vi "Write Startup Model-View Configuration.vi"(8 "Mediator":refnum<class "IMediator.lvclass">, 9 "Model":refnum<class "IModel.lvclass">, 10 "Startup View Configuration":refnum<class "IViewable.lvclass">, 11 "IViewModel In":refnum<class "IViewModel.lvclass">) -> (3 "IViewModel Out":refnum<class "IViewModel.lvclass">)   [LabVIEW 2015, in "IViewModel.lvlib" / "IViewModel.lvclass"]
doc: "<License>\nCopyright © 2017 Composed Systems, LLC | All rights reserved\nwww.composed.io\n\nAuthor: Ethan Stern <ethan.stern@composed.io>\n\nThis software is provided \"AS IS\" WITHOUT WARRANTIES, either express or implied, AND IS FOR EDUCATIONAL PURPOSES ONLY.\n</License>"
uses:
  IViewModel.lvclass
  IViewable/IViewable/IViewable.lvclass
  IModel/IModel/IModel.lvclass
  IMediator/IMediator/IMediator.lvclass
  IViewModel.lvclass/IViewModel.ctl
  IViewManager/IViewManager Messages/Launch Nested Views Msg/Launch Nested Views Msg.lvclass/Launch Nested Views Msg.ctl
  IViewManager/IViewManager/IViewManager.lvclass/IViewManager.ctl
  IViewManager/IViewManager Messages/Launch Nested Views Msg/Launch Nested Views Msg.lvclass
  IViewManager/IViewManager/IViewManager.lvclass
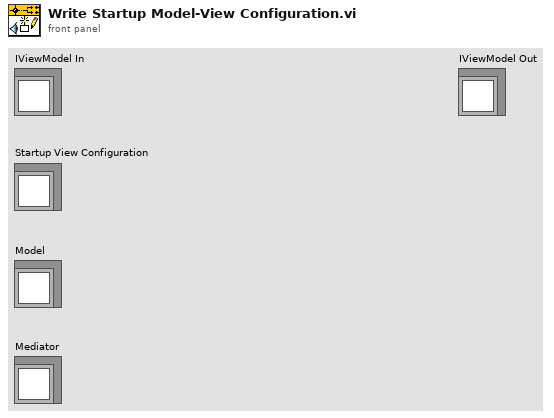
[diagram p1: front panel]
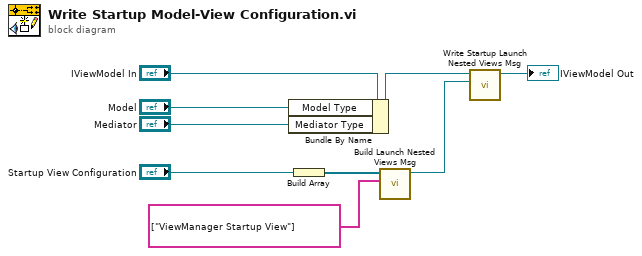
[diagram p0: block diagram]
diagram:
  n1 = Bundle By Name(cluster="IViewModel In", "Model Type"="Model", "Mediator Type"="Mediator") -> (w3:refnum<class "IViewModel.lvclass">)
  n2 = Build Array("Startup View Configuration") -> (w7:refnum<class "IViewable.lvclass">[])
  n3 = call "Build Launch Nested Views Msg.vi"("View Labels"=string[] ["ViewManager Startup View"] ("View Labels (optional)"), "Nested Views"=w7) -> ("Launch Nested Views Msg out"=w5:refnum<class "Launch Nested Views Msg.lvclass">)  [unwired: 8 in, 1 out]
  n4 = call "Write Startup Launch Nested Views Msg.vi"("Launch Nested Views Msg"=w5, "IViewManager in"=w3) -> ("IViewManager out"=→"IViewModel Out":refnum<class "IViewModel.lvclass">)  [unwired: 8 in, 1 out]
